vi "CloseSink.vi"(8 "error in (no error)":errorcluster, 11 "RelayAppender in":refnum<class "RelayAppender.lvclass">) -> (0 "error out":errorcluster, 3 "RelayAppender out":refnum<class "RelayAppender.lvclass">)   [LabVIEW 2026, in "Lumberjack.lvlib" / "RelayAppender.lvclass"]
doc: "Flush and close this appender's sink resource. Called once on actor exit (from Actor Core), including the error-exit path, so buffered data is not lost on shutdown. Abstract: each concrete appender closes its own sink. DD, must override."
uses:
  RelayAppender.lvclass
  RelayAppender.lvclass/RelayAppender.ctl
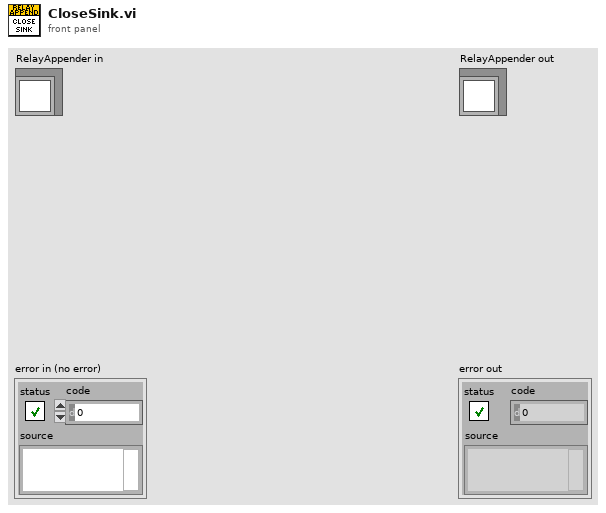
[diagram p1: front panel]
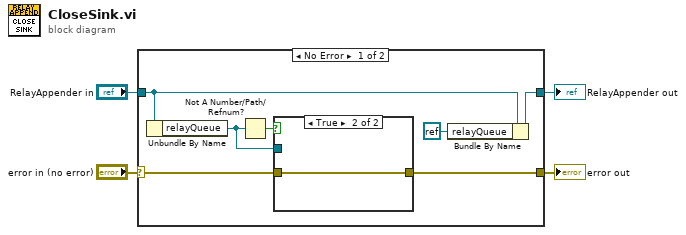
[diagram p0: block diagram]
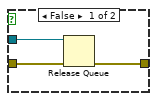
[diagram p2: hidden frame]
diagram:
  n1 = case shown="No Error" "error in (no error)" {
    selector: "error in (no error)" -> [w11 w17]
    tunnel: [w10 w17] -> w4
    tunnel: [w5 w16] -> w3
    tunnel: "RelayAppender in" -> [w6 w16]
    frame No Error {
      n2 = Unbundle By Name(w6) -> ("relayQueue"=w8:refnum<queue>)
      n3 = Not A Number/Path/Refnum?(number/path/refnum=w8) -> (NaN/Path/Refnum?=w9:bool)
      n4 = case shown="True" w9 {
        tunnel: w11 -> [w14 w15]
        tunnel: [w13 w15] -> w10
        tunnel: w8 -> [w12 _]
        frame False {
          n5 = Release Queue(queue=w12, error in (no error)=w14) -> (error out=w13:errorcluster)  [unwired: 1 in, 2 out]
        }
        frame True {
        }
      }
      n6 = Bundle By Name(cluster=w6, "relayQueue"=refnum<k0> refnum) -> (w5:refnum<class "RelayAppender.lvclass">)
    }
    frame Error {
    }
  }
  "error out" <- w4
  "RelayAppender out" <- w3
